vi "CreatePrivateEvents.vi"(8 "error in (no error)":errorcluster, 11 "RemoteControl":refnum<class "RemoteControl.lvclass">) -> (0 "error out":errorcluster, 3 "RemoteControl out":refnum<class "RemoteControl.lvclass">)   [LabVIEW 2020, in "RemoteControl.lvclass"]
doc: "---------------------------------------------------------------\nJKI State Machine Objects™\nhttp://jki.net/state-machine-objects/\nCopyright (C) 2005-2015, JKI <info@jki.net>\nALL RIGHTS RESERVEDJKI State Machine Objects (SMO) 1.0.0.4\nJKI - JKI\nCopyright (c) 2015, JKI"
uses:
  RemoteControl.lvclass
  Typedefs/PrivateEvents--RemoteControl.Configure.ctl
  Typedefs/PrivateEvents--RemoteControl.SendMessageToProcess.ctl
  Typedefs/Message--Cluster.ctl
  RemoteControl.lvclass/RemoteControl.ctl
  LevyLab/LevyLab.lvclass
panel:
  # "For instructions on how to use the JKI State Machine Objects, examples and video tutorials, visit:\nhttp://jki.net/state-machine-objects/\n\nJKI State Machine Objects™\nhttp://jki.net/state-machine-objects/\nCopyright (C) 2005-2015, JKI <info@jki.net>\nALL RIGHTS RESERVED"
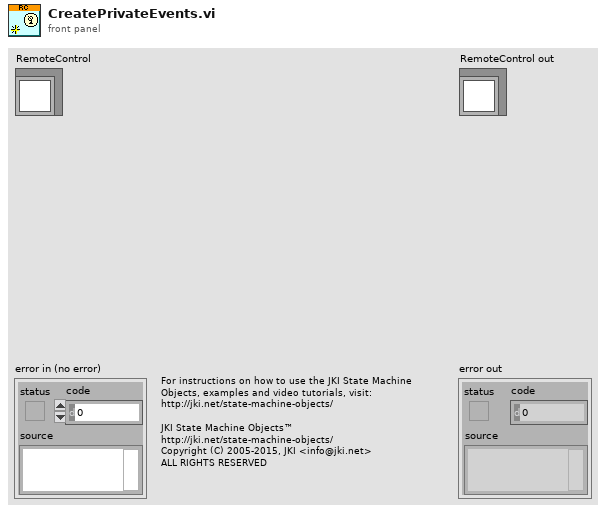
[diagram p1: front panel]
types:
  T1 = typedef "RemoteControl.lvclass/PrivateEvents--RemoteControl.SendMessageToProcess.ctl" = cluster{"Message":T2}
  T2 = typedef "RemoteControl.lvclass/Message--Cluster.ctl" = cluster{"Command":string, "Data":variant, "Message ID":i32}
  T3 = typedef "RemoteControl.lvclass/PrivateEvents--RemoteControl.Configure.ctl" = cluster{"address":string, "Port":u16, "AllowedRemote":string, "Commands":string[]}
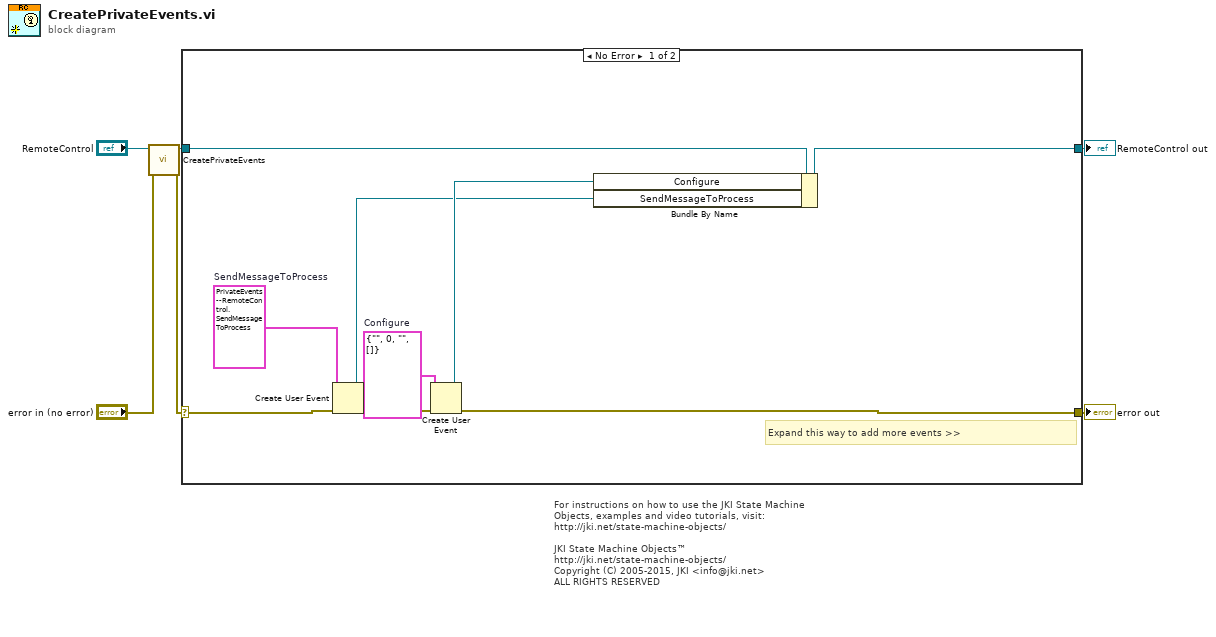
[diagram p0: block diagram]
diagram:
  # "For instructions on how to use the JKI State Machine Objects, examples and video tutorials, visit:\nhttp://jki.net/state-machine-objects/\n\nJKI State Machine Objects™\nhttp://jki.net/state-machine-objects/\nCopyright (C) 2005-2015, JKI <info@jki.net>\nALL RIGHTS RESERVED"
  n1 = call-parent "CreatePrivateEvents.vi"("error in (no error)"="error in (no error)", "SMO"="RemoteControl") -> ("error out"=w1:errorcluster, "SMO out"=w3:refnum<class "RemoteControl.lvclass">)  [unwired: 8 in]
  n2 = case shown="No Error" w1 {
    selector: w1 -> [w14 w17]
    tunnel: [w7 w17] -> w5
    tunnel: [w13 w16] -> w6
    tunnel: w3 -> [w15 w16]
    frame No Error {
      w9 = T1 {"Message"={"Command"="", "Data"=variant(bool FALSE), "Message ID"=0}}  # SendMessageToProcess
      w12 = T3 {"address"="", "Port"=0, "AllowedRemote"="", "Commands"=[]}  # Configure
      # "Expand this way to add more events >>"
      n3 = Create User Event(user event datatype=w9, error in=w14) -> (user event=w8:refnum<user-event>, error out=w10:errorcluster)
      n4 = Create User Event(user event datatype=w12, error in=w10) -> (user event=w11:refnum<user-event>, error out=w7:errorcluster)
      n5 = Bundle By Name(cluster=w15, "Configure"=w11, "SendMessageToProcess"=w8) -> (w13:refnum<class "RemoteControl.lvclass">)
    }
    frame Error {
    }
  }
  "error out" <- w5
  "RemoteControl out" <- w6
